vi "onRemoveHeaders.vi"(8 "error in (no error)":errorcluster, 10 "headers (empty: all)":string[](array[string]), 11 "httpHeaders in":refnum<class "httpHeaders.lvclass">) -> (0 "error out":errorcluster, 3 "httpHeaders out":refnum<class "httpHeaders.lvclass">)   [LabVIEW 2020, in "httpClient.lvlib" / "httpHeaders.lvclass"]
uses:
  httpHeaders.lvclass
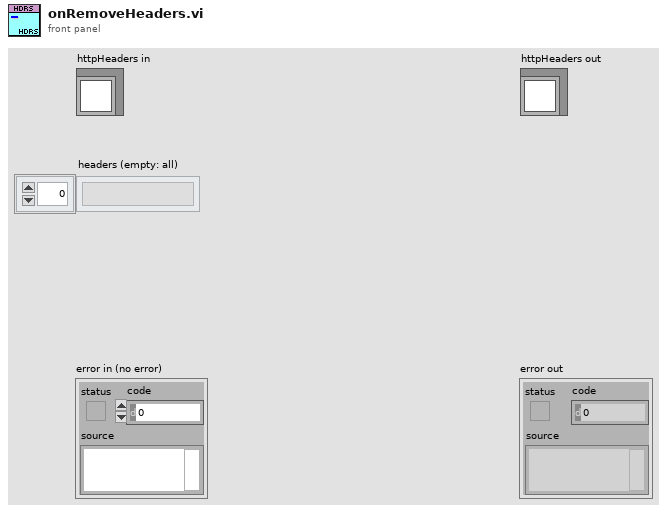
[diagram p1: front panel]
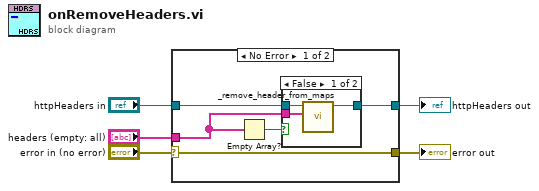
[diagram p0: block diagram]
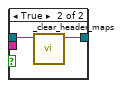
[diagram p2: hidden frame]
diagram:
  n1 = case shown="No Error" "error in (no error)" {
    selector: "error in (no error)" -> [w10 w17]
    tunnel: [w10 w17] -> w4
    tunnel: [w8 w16] -> w2
    tunnel: "httpHeaders in" -> [w9 w16]
    tunnel: "headers (empty: all)" -> [w6 _]
    frame No Error {
      n2 = Empty Array?(array=w6) -> (empty?=w7:bool)
      n3 = case shown="False" w7 {
        tunnel: w9 -> [w13 w15]
        tunnel: [w12 w14] -> w8
        tunnel: w6 -> [w11 _]
        frame False {
          n4 = call "_remove_header_from_maps.vi"("header"=w11, "httpHeaders in"=w13) -> ("httpHeaders out"=w12:refnum<class "httpHeaders.lvclass">)  [unwired: 9 in]
        }
        frame True {
          n5 = call "_clear_header_maps.vi"("httpHeaders in"=w15) -> ("httpHeaders out"=w14:refnum<class "httpHeaders.lvclass">)  [unwired: 10 in]
        }
      }
    }
    frame Error {
    }
  }
  "error out" <- w4
  "httpHeaders out" <- w2
